vi "Calibration Alert.vi"(8 "error in (no error)":errorcluster, 11 "message":string) -> (0 "error out":errorcluster)   [LabVIEW 2020]
doc: "Displays a standard dialog box that prompts users to enter information, such as a user name and password.\n--------------------\n\nThis Express VI is configured as follows:\n\nMessage to Display to the User:\nThe inputs are:"
panel:
  out "message 2":string
  in  "quit":bool caption="Cancel"
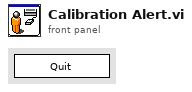
[diagram p1: front panel]
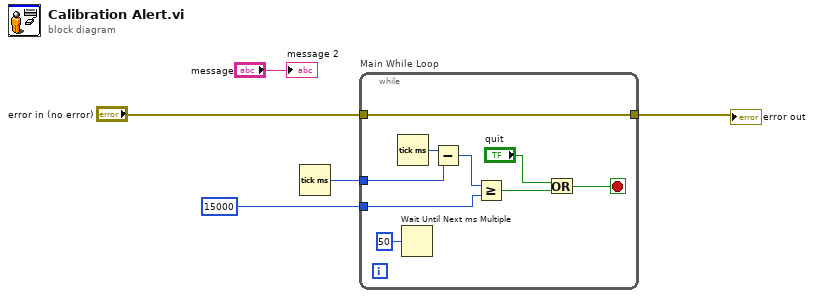
[diagram p0: block diagram]
diagram:
  n1 = Tick Count (ms)() -> (millisecond timer value=w5:u32)
  n2 = while "Main While Loop" {
    tunnel: "error in (no error)" -> [w12]
    tunnel: [w12] -> w2
    tunnel: w5 -> [w9]
    tunnel: u32 15000 ("timeout, msec (5000)") -> [w8]
    stop <- w6 stop-if-true
    n3 = Tick Count (ms)() -> (millisecond timer value=w11:u32)
    n4 = Wait Until Next ms Multiple(millisecond multiple=u32 50) -> ()  [unwired: 1 out]
    n5 = Subtract(x=w11, y=w9) -> (x-y=w10:u32)
    n6 = Greater Or Equal?(x=w10, y=w8) -> (x >= y?=w7:bool)
    n7 = Or(x="quit", y=w7) -> (x .or. y?=w6:bool)
  }
  "error out" <- w2
  "message 2" <- "message"
